vi "Turn Blocker.vi"(1 "Run?":bool) -> ()   [LabVIEW 2013]
uses:
  Globals/Useful Values.vi
panel:
  out "Vision Turn":dbl
  out "Done?":bool
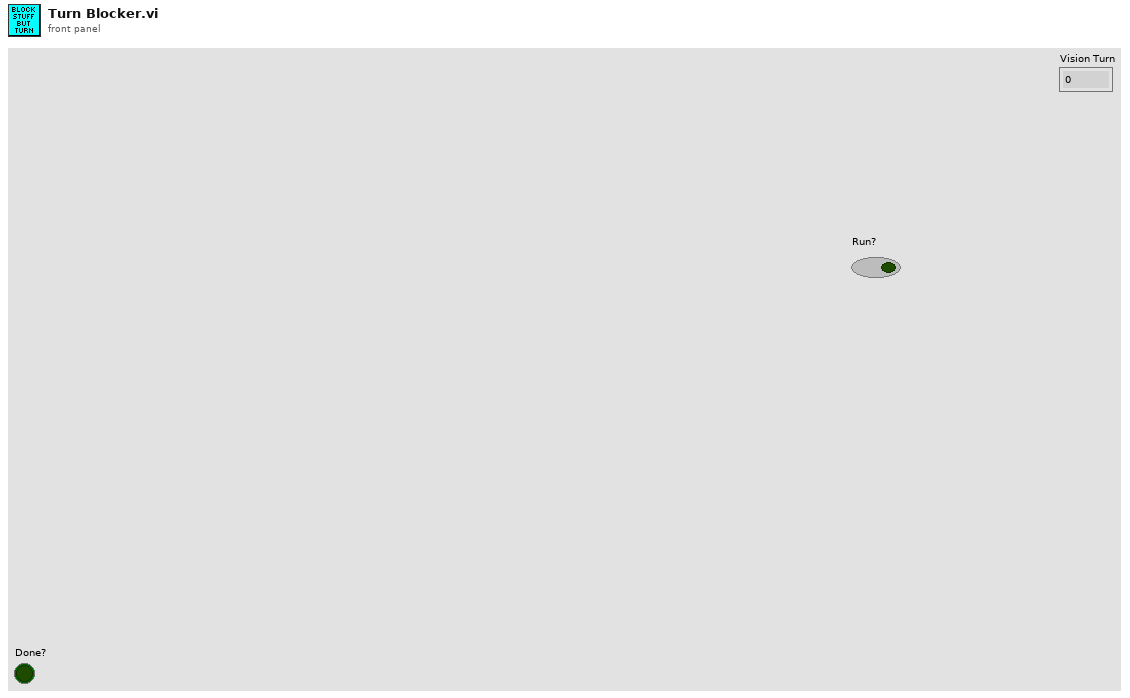
[diagram p1: front panel]
types:
  T1 = typedef "WPI_AnalogChannelDevRef.ctl" = cluster{"DevStatus":errorcluster, "Analog Module":T2, "Analog Channel":T3}
  T2 = typedef "FPGA_TypedefAnalogModule.ctl" = enum16{"Analog Module 1", "Analog Module 2"}
  T3 = typedef "FPGA_AIChannel.ctl" = enum8{"AI 1", "AI 2", "AI 3", "AI 4", "AI 5", "AI 6", "AI 7", "AI 8", "Invalid"}
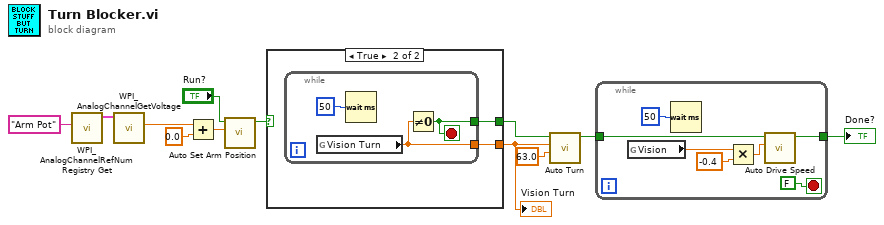
[diagram p0: block diagram]
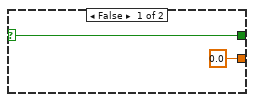
[diagram p2: hidden frame]
diagram:
  n1 = call <vilib>:"WPI_AnalogChannelRefNum Registry Get.vi"("refnum name"="Arm Pot") -> ("AIDeviceRef"=w9:T1)  [unwired: 9 in, 1 out]
  n2 = call <vilib>:"WPI_AnalogChannelGetVoltage.vi"("AIDeviceRef"=w9) -> ("Voltage"=w7:dbl)  [unwired: 8 in, 2 out]
  n3 = Add(x=w7, y=0.0) -> (x+y=w2:dbl)
  n4 = call "Auto Set Arm Position.vi"("Arm Position"=w2, "Run?"="Run?") -> ("Done"=w5:bool)  [unwired: 9 in]
  n5 = case shown="True" w5 {
    selector: w5 -> [w14 _]
    tunnel: [0.0 ("Vision Turn") w16] -> w11
    tunnel: [w14 w15] -> w10
    frame False {
    }
    frame True {
      n6 = while {
        tunnel: [w18] -> w16
        tunnel: [w17] -> w15
        stop <- w17 stop-if-true
        n7 = global read "Useful Values.vi" "Vision Turn"() -> (w18:dbl)
        n8 = Wait (ms)(milliseconds to wait=u32 50) -> ()  [unwired: 1 out]
        n9 = Not Equal To 0?(x=w18) -> (x != 0?=w17:bool)
      }
    }
  }
  "Vision Turn" <- w11
  n10 = call "Auto Turn.vi"("Turn Amount"=63.0, "+/-?"=w11, "Run?"=w10) -> ("Done"=w3:bool)  [unwired: 8 in]
  n11 = while {
    tunnel: [w22] -> w4
    tunnel: w3 -> [w20]
    stop <- FALSE stop-if-true
    n12 = global read "Useful Values.vi" "Vision"() -> (w24:dbl)
    n13 = Wait (ms)(milliseconds to wait=u32 50) -> ()  [unwired: 1 out]
    n14 = Multiply(x=w24, y=-0.4) -> (x*y=w23:dbl)
    n15 = call "Auto Drive Speed.vi"("Output"=w23, "Run?"=w20) -> ("Done"=w22:bool)  [unwired: 9 in]
  }
  "Done?" <- w4
